vi "_Electronic On.vi"   [LabVIEW 2012]
uses:
  <vilib>/rvi/DataTransferAndStorage/Container/Common/niFpgaContainerGetUniqueNameForEmu.vi
  <vilib>/rvi/Memory/Memory_Emulation/niFpgaMemoryEmulationCacheClearOnFirstRun.vi
  <vilib>/rvi/Memory/Memory_Emulation/nirvimemoryEmulationManagerCache_MakeExclusive.vi
  <vilib>/rvi/Memory/Memory_Emulation/niFpgaMemoryEmulationValidateCache.vi
  <vilib>/rvi/Memory/Memory_Emulation/nirvimemoryEmulationManagerCache_ReleaseExclusive.vi
  <vilib>/rvi/Memory/Memory_Emulation/nirvimemoryEmulationManagerCache_InsertValue.vi
  <vilib>/Utility/error.llb/Clear Errors.vi
  <vilib>/rvi/Memory/Memory_Emulation/nirvimemoryEmulationManagerCache_GetValue.vi
  <vilib>/rvi/eio/common/nirviEmuTemplateMethod_errors.vi
  <vilib>/rvi/DataTransferAndStorage/Container/XNode/niFpgaContainer.xnode
  <vilib>/rvi/Memory/Memory_Emulation/nirvimemoryEmulation.vi
  <vilib>/eio/EIONode/EIONode.xnode
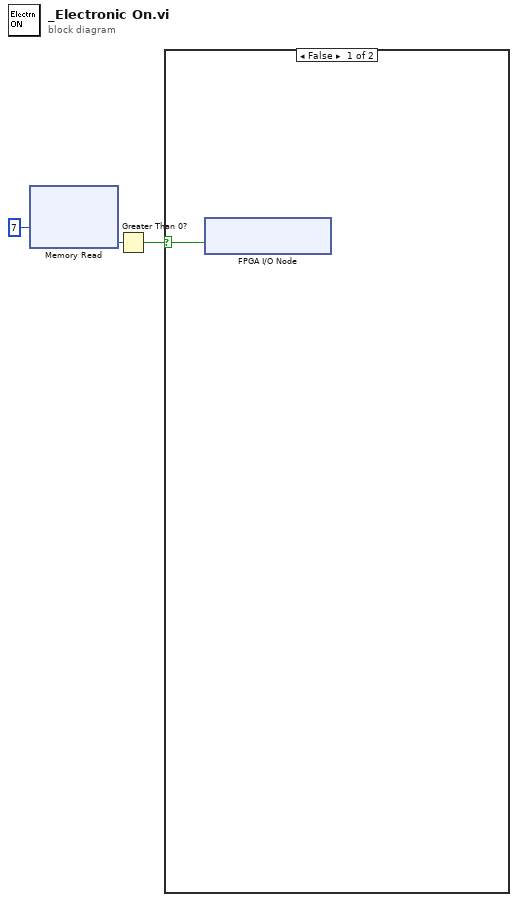
[diagram p0: block diagram]
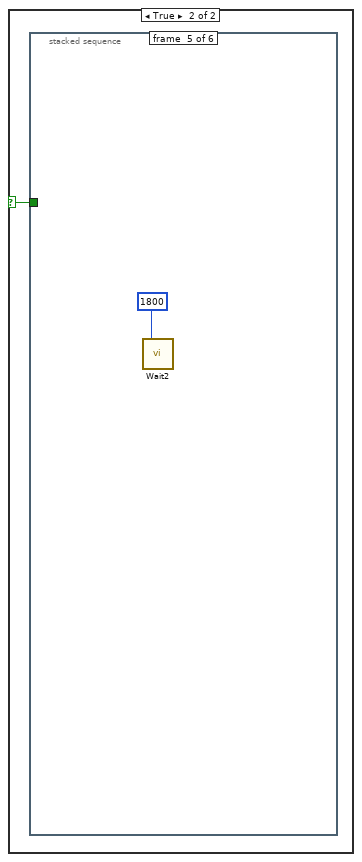
[diagram p2: hidden frame]
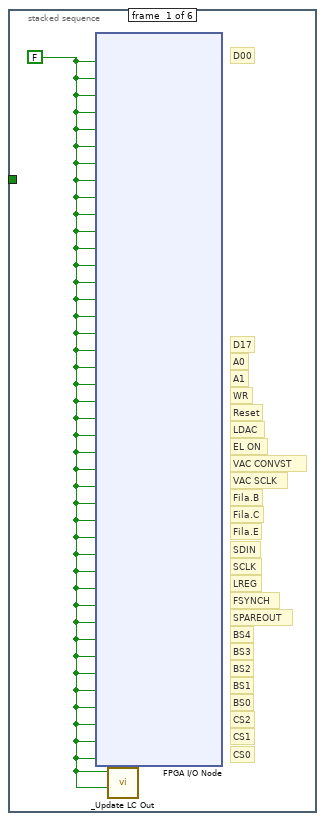
[diagram p3: hidden frame]
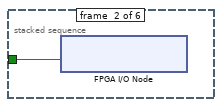
[diagram p4: hidden frame]
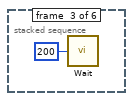
[diagram p5: hidden frame]
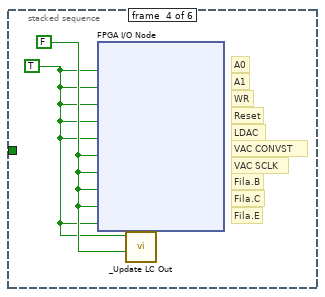
[diagram p6: hidden frame]
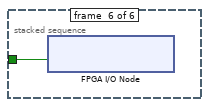
[diagram p7: hidden frame]
diagram:
  n1 = xnode ("Memory Read")("Address"=u8 7) -> ("Data"=w3:u32)  [unwired: 1 in, 1 out]
  n2 = Greater Than 0?(x=w3) -> (x > 0?=w1:bool)
  n3 = case shown="False" w1 {
    selector: w1 -> [w4 w5]
    frame False {
      n4 = xnode "FPGA I/O Node"("Digtal IO/DIO23"=w4) -> ()  [unwired: 1 in, 1 out]
    }
    frame True {
      n5 = stacked-sequence {
        tunnel: w5 -> [_ w7 _ _ _ w12]
        frame #0 {
          w6 = FALSE ("Port4/DIO8")
          # "CS0"
          # "CS1"
          # "CS2"
          # "BS0"
          # "BS1"
          # "BS2"
          # "BS3"
          # "BS4"
          # "SPAREOUT"
          # "FSYNCH"
          # "LREG"
          # "SCLK"
          # "SDIN"
          # "Fila.E"
          # "Fila.C"
          # "Fila.B"
          # "VAC SCLK"
          # "VAC CONVST"
          # "EL ON"
          # "LDAC"
          # "WR"
          # "A1"
          # "A0"
          # "Reset"
          # "D17"
          # "D00"
          n6 = xnode "FPGA I/O Node"("Digtal IO/DIO42"=w6, "Digtal IO/DIO41"=w6, "Digtal IO/DIO40"=w6, "Digtal IO/DIO39"=w6, "Digtal IO/DIO38"=w6, "Digtal IO/DIO37"=w6, "Digtal IO/DIO36"=w6, "Digtal IO/DIO35"=w6, "Digtal IO/DIO34"=w6, "Digtal IO/DIO32"=w6, "Digtal IO/DIO31"=w6, "Digtal IO/DIO30"=w6, "Digtal IO/DIO29"=w6, "Digtal IO/DIO28"=w6, "Digtal IO/DIO27"=w6, "Digtal IO/DIO26"=w6, "Digtal IO/DIO25"=w6, "Digtal IO/DIO24"=w6, "Digtal IO/DIO62"=w6, "Digtal IO/DIO61"=w6, "Digtal IO/DIO64"=w6, "Digtal IO/DIO13"=w6, "Digtal IO/DIO63"=w6, "Digtal IO/DIO23"=w6, "Digtal IO/DIO57"=w6, "Digtal IO/DIO58"=w6, "Digtal IO/DIO66"=w6, "Digtal IO/DIO67"=w6, "Digtal IO/DIO68"=w6, "Digtal IO/DIO8"=w6, "Digtal IO/DIO9"=w6, "Digtal IO/DIO10"=w6, "Digtal IO/DIO11"=w6, "Digtal IO/DIO12"=w6, "Digtal IO/DIO14"=w6, "Digtal IO/DIO15"=w6, "Digtal IO/DIO16"=w6, "Digtal IO/DIO17"=w6, "Digtal IO/DIO19"=w6, "Digtal IO/DIO20"=w6, "Digtal IO/DIO21"=w6, "Digtal IO/DIO22"=w6) -> ()  [unwired: 42 in, 42 out]
          n7 = call "_Update LC Out.vi"("LC Stop"=w6, "LC Hold"=w6) -> ()  [unwired: 6 out]
        }
        frame #1 {
          n8 = xnode "FPGA I/O Node"("Digtal IO/DIO23"=w7) -> ()  [unwired: 1 in, 1 out]
        }
        frame #2 {
          n9 = call "Wait"("Count(mSec)"=u8 200) -> ()  [unwired: 1 out]
        }
        frame #3 {
          w9 = TRUE
          w10 = FALSE ("Port4/DIO8")
          # "Fila.E"
          # "Fila.C"
          # "Fila.B"
          # "VAC SCLK"
          # "VAC CONVST"
          # "LDAC"
          # "WR"
          # "A1"
          # "A0"
          # "Reset"
          n10 = xnode "FPGA I/O Node"("Digtal IO/DIO62"=w9, "Digtal IO/DIO61"=w9, "Digtal IO/DIO64"=w9, "Digtal IO/DIO13"=w9, "Digtal IO/DIO63"=w9, "Digtal IO/DIO57"=w10, "Digtal IO/DIO58"=w10, "Digtal IO/DIO66"=w10, "Digtal IO/DIO67"=w10, "Digtal IO/DIO68"=w9) -> ()  [unwired: 10 in, 10 out]
          n11 = call "_Update LC Out.vi"("LC Stop"=w10, "LC Hold"=w9) -> ()  [unwired: 6 out]
        }
        frame #4 {
          n12 = call "Wait2"("Count(mSec)"=u16 1800) -> ()  [unwired: 1 out]
        }
        frame #5 {
          n13 = xnode "FPGA I/O Node"("Digtal IO/DIO57"=w12) -> ()  [unwired: 1 in, 1 out]
        }
      }
    }
  }
